vi "Is Step in Range.vi"(9 "Array Size":i32, 11 "Chosen Step":dbl) -> (2 "In Range?":bool, 3 "Index out":i32)   [LabVIEW 2021]
doc: "Determines if <B>Chosen Step</B> is less than or equal to <B>Array Size</B>."
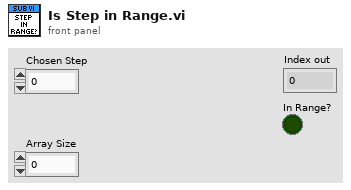
[diagram p1: front panel]
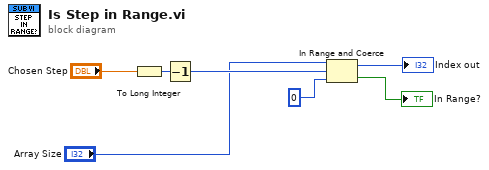
[diagram p0: block diagram]
diagram:
  n1 = To Long Integer(number="Chosen Step") -> (32bit integer=w6:i32)
  n2 = Decrement(x=w6) -> (x-1=w5:i32)
  n3 = In Range and Coerce(upper limit="Array Size", x=w5, lower limit=0) -> (coerced(x)=→"Index out":i32, In Range?=→"In Range?":bool)
